vi "connect_group.vi"(2 "Имя группы":string, 3 "JSON":string) -> (0 "error out":errorcluster)   [LabVIEW 2022 SP3]
panel:
  # "Получает JSON проекта и имя группы которую нужно скомутировать и посылает \nкоманды коммутации на матрицу.\nПеред комутацией происходит анализ текущих коммутаций и отключение только тех реле которые больше не нужны (сохранение ресурса реле)"
  # "СТРОКА JSON {groups:[{комутация1},{комутация2},{комутация3},...], matrixs:[имя матицы1, имя матрицы2,...]}\n{комутация} - это {\"name\": имя коммутации, \"code\":[[точка],[точка],...]}\nнапример {\"groups\": [{\"name\": \"тестовая\", \"code\": [[\"c43\", \"r0\", \"эталоны\"],..., \"matrixs\": [\"эталоны\", \"Сторона_А\"..."
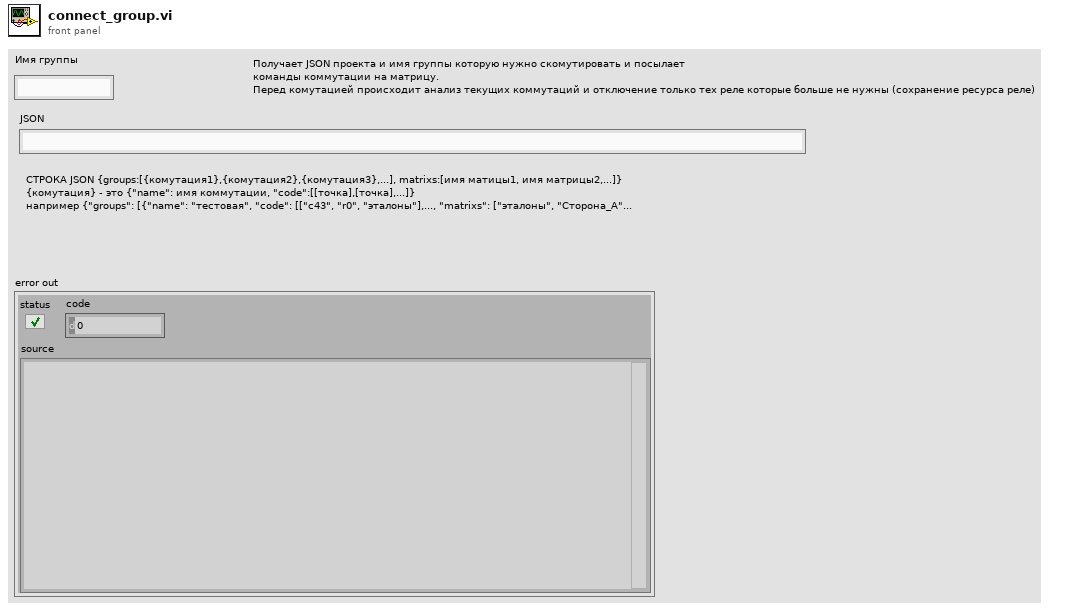
[diagram p1: front panel]
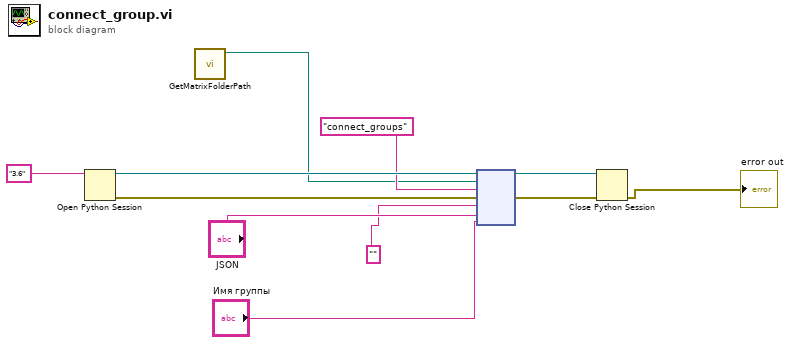
[diagram p0: block diagram]
diagram:
  n1 = Open Python Session(python version="3.6" ("Python version")) -> (session out=w6:refnum<k35>, error out=w7:errorcluster)  [unwired: 2 in]
  n2 = call "GetMatrixFolderPath.vi"() -> ("module path"=w1:path)  [unwired: 11 in]
  n3 = node(w6, w1, "connect_groups" ("function name"), w7, "", "JSON", "Имя группы") -> (w10:refnum<k35>, w9:errorcluster)  [unwired: 3 in, 2 out]
  n4 = Close Python Session(session in=w10, error in=w9) -> (11:→"error out":errorcluster)
